vi "Wire Defaults.vi"(6 "Names":string[](array[string]), 8 "error in (no error)":errorcluster, 10 "SubVI Outputs":refnum<vi>[](array[refnum]), 11 "VI in":refnum<vi>) -> (0 "error out":errorcluster, 3 "VI":refnum<vi>)   [LabVIEW 2020, in "Conditum-Tools.lvlib" / "Entity Editor.lvclass"]
uses:
  Entity Editor.lvclass
  <vilib>/Utility/traverseref.llb/TRef TravTarget.ctl
  <vilib>/Utility/traverseref.llb/VI Scripting - Traverse.lvlib
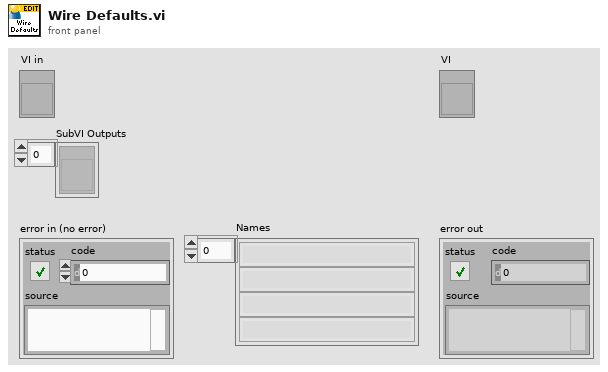
[diagram p1: front panel]
types:
  T1 = typedef "TRef TravTarget.ctl" = enum16{"FP", "BD", "Other"}
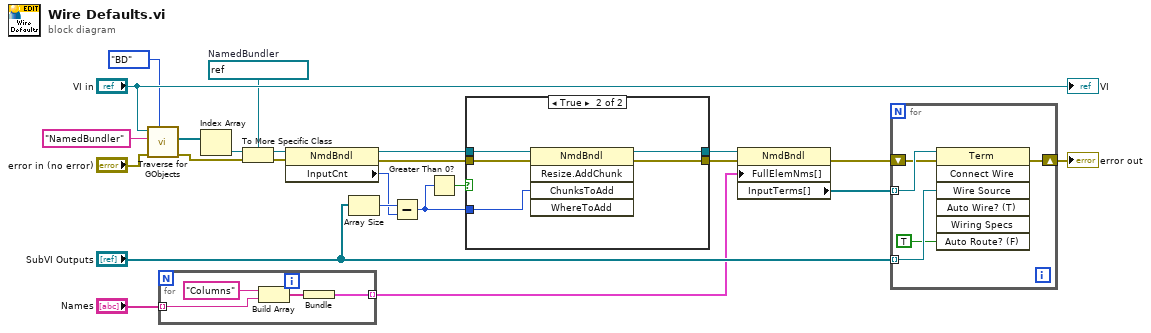
[diagram p0: block diagram]
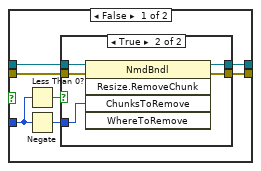
[diagram p2: hidden frame]
diagram:
  w19 = refnum<vi> refnum  # NamedBundler
  n1 = call <vilib>:"Traverse for GObjects.vi"("Traverse Target"=TRef_TravTarget."BD", "error in (no error)"="error in (no error)", "Class Name"="NamedBundler", "VI Refnum"="VI in") -> ("error out"=w11:errorcluster, "References"=w21:refnum<vi>[])  [unwired: 4 in, 2 out]
  n2 = for {
    tunnel: "Names" -> [w27] mode=indexing
    tunnel: [w25] -> w1 mode=indexing
    n3 = Build Array("Columns" ("string"), w27) -> (w26:string[])
    n4 = Bundle(w26) -> (w25:cluster{string[]})  [unwired: 1 in]
  }
  n5 = Index Array(array=w21) -> (element=w20:refnum<vi>)  [unwired: 1 in]
  n6 = To More Specific Class(target class=w19, reference=w20, error in=w11) -> (specific class reference=w18:refnum<vi>, error out=w17:errorcluster)
  n7 = property class="NmdBndl"(reference=w18, error in=w17) -> (reference out=w14:refnum<vi>, error out=w9:errorcluster, "InputCnt"=w15:i32)
  n8 = Array Size(array="SubVI Outputs") -> (size(s)=w16:i32)
  n9 = Subtract(x=w16, y=w15) -> (x-y=w12:i32)
  n10 = Greater Than 0?(x=w12) -> (x > 0?=w13:bool)
  n11 = case shown="True" w13 {
    tunnel: w14 -> [w34 w47]
    tunnel: w12 -> [w35 w46]
    tunnel: [w30 w45] -> w8
    tunnel: w9 -> [w33 w44]
    tunnel: [w29 w43] -> w7
    frame False {
      n12 = Less Than 0?(x=w35) -> (x < 0?=w32:bool)
      n13 = Negate(x=w35) -> (-x=w31:i32)
      n14 = case shown="True" w32 {
        tunnel: w34 -> [w37 w42]
        tunnel: w33 -> [w36 w41]
        tunnel: w31 -> [_ w40]
        tunnel: [w37 w39] -> w30
        tunnel: [w36 w38] -> w29
        frame False {
        }
        frame True {
          n15 = invoke class="NmdBndl" method="Resize.RemoveChunk"(reference=w42, error in=w41, "ChunksToRemove"=w40) -> (reference out=w39:refnum<vi>, error out=w38:errorcluster)  [unwired: 2 in, 3 out]
        }
      }
    }
    frame True {
      n16 = invoke class="NmdBndl" method="Resize.AddChunk"(reference=w47, error in=w44, "ChunksToAdd"=w46) -> (reference out=w45:refnum<vi>, error out=w43:errorcluster)  [unwired: 2 in, 3 out]
    }
  }
  n17 = property class="NmdBndl"(reference=w8, error in=w7, "FullElemNms[]"=w1) -> (error out=w6:errorcluster, "InputTerms[]"=w4:refnum<vi>[])  [unwired: 1 out]
  n18 = for {
    shift-right: [w50] -> w3
    shift-left: w6 -> [w51]
    tunnel: "SubVI Outputs" -> [w49] mode=indexing
    tunnel: w4 -> [w52] mode=indexing
    n19 = invoke class="Term" method="Connect Wire"(reference=w52, error in=w51, "Wire Source"=w49, "Auto Route? (F)"=TRUE) -> (error out=w50:errorcluster)  [unwired: 3 in, 6 out]
  }
  "error out" <- w3
  "VI" <- "VI in"
